vi "Get Oblique Correction.vi"(10 "Mean Obique Ecliptic Longitude":dbl, 11 "Julian Century":dbl) -> (3 "Oblique Correction (deg)":dbl)   [LabVIEW 2014, in "Solar Calculations.lvlib"]
uses:
  Solar Calculations.lvlib
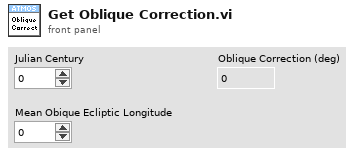
[diagram p1: front panel]
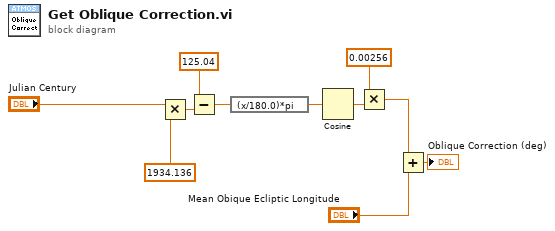
[diagram p0: block diagram]
diagram:
  n1 = Multiply(x="Julian Century", y=1934.136) -> (x*y=w4:dbl)
  n2 = Subtract(x=125.04, y=w4) -> (x-y=w6:dbl)
  n3 = expression code="(x/180.0)*pi" ("degrees to radians")(w6) -> (w7:dbl)
  n4 = Cosine(x=w7) -> (cos(x)=w8:dbl)
  n5 = Multiply(x=0.00256, y=w8) -> (x*y=w10:dbl)
  n6 = Add(x=w10, y="Mean Obique Ecliptic Longitude") -> (x+y=→"Oblique Correction (deg)":dbl)
